vi "Save_to_Project.vi"(8 "error in (no error)":errorcluster, 9 "index in":string, 10 "buildObject":T2, 11 "IB_RegGroup in":refnum<class "IB_RegGroup.lvclass">) -> (0 "error out":errorcluster, 1 "index out":string, 2 "buildObject out":T2, 3 "IB_RegGroup out":refnum<class "IB_RegGroup.lvclass">)   [LabVIEW 2020, in "IB_RegGroup.lvclass"]
uses:
  <vilib>/AppBuilder/IB_Classes/RegGroup/IB_RegGroup.lvclass
  <vilib>/AppBuilder/IB_Classes/RegGroup/IB_RegGroup.lvclass/IB_RegGroup.ctl
  <vilib>/AppBuilder/IB_Classes/RegData/IB_RegData.lvclass
  <vilib>/AppBuilder/IB_RW_Project/IB_RW_Project_PropBag_Action.ctl
  <resource>/Framework/Providers/API/ItemRef.ctl
  <vilib>/AppBuilder/IB_RW_Project/IB_RW_Project_RegGroup_Data.ctl
panel:
  in  "RegGroup":T1
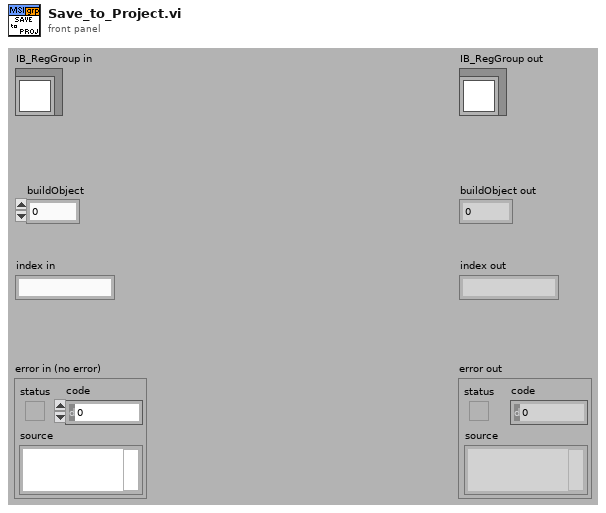
[diagram p1: front panel]
types:
  T1 = typedef "IB_RW_Project_RegGroup_Data.ctl" = cluster{"dirTag":string}
  T2 = typedef "ItemRef.ctl" = u64
  T3 = typedef "IB_RW_Project_PropBag_Action.ctl" = enum16{"read", "write", "clear", "readPrevious", "writePrevious", "clearPrevious"}
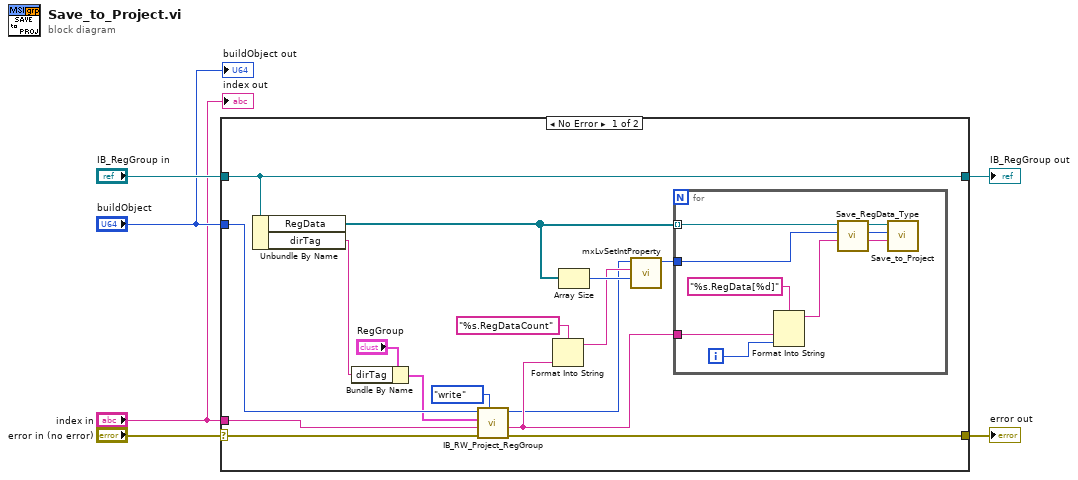
[diagram p0: block diagram]
diagram:
  n1 = case shown="No Error" "error in (no error)" {
    selector: "error in (no error)" -> [w16 w33]
    tunnel: [w15 w33] -> w5
    tunnel: [w18 w32] -> w3
    tunnel: "IB_RegGroup in" -> [w18 w32]
    tunnel: "buildObject" -> [w13 _]
    tunnel: "index in" -> [w12 _]
    frame No Error {
      n2 = Unbundle By Name(w18) -> ("RegData"=w17:refnum<class "IB_RegData.lvclass">[], "dirTag"=w8:string)
      n3 = Bundle By Name(cluster="RegGroup", "dirTag"=w8) -> (w7:T1)
      n4 = call <vilib>:"IB_RW_Project_RegGroup.vi"("action"=IB_RW_Project_PropBag_Action."write", "error in (no error)"=w16, "index in"=w12, "RegGroup"=w7, "buildObject"=w13) -> ("error out"=w15:errorcluster, "index out"=w11:string, "buildObject out"=w10:T2)  [unwired: 3 in, 1 out]
      n5 = Format Into String(format string="%s.RegDataCount", w11) -> (resulting string=w21:string)  [unwired: 2 in, 1 out]
      n6 = Array Size(array=w17) -> (size(s)=w22:i32)
      n7 = call <resource>:"mxLvSetIntProperty.vi"("Value (0)"=w22, "Tag"=w21, "Item"=w10) -> ("Item"=w19:T2)  [unwired: 7 in, 1 out]
      n8 = for {
        tunnel: w17 -> [w28] mode=indexing
        tunnel: w19 -> [w26]
        tunnel: w11 -> [w30]
        i -> [w29]
        n9 = Format Into String(format string="%s.RegData[%d]", w30, w29) -> (resulting string=w24:string)  [unwired: 2 in, 1 out]
        n10 = call-dynamic "Save_RegData_Type.vi"("index in"=w24, "buildObject"=w26, "IB_RegData in"=w28) -> ("index out"=w23:string, "buildObject out"=w25:T2, "IB_RegData out"=w27:refnum<class "IB_RegData.lvclass">)  [unwired: 5 in, 1 out]
        n11 = call-dynamic "Save_to_Project.vi"("index in"=w23, "buildObject"=w25, "IB_RegData in"=w27) -> ()  [unwired: 5 in, 4 out]
      }
    }
    frame Error {
    }
  }
  "error out" <- w5
  "IB_RegGroup out" <- w3
  "buildObject out" <- "buildObject"
  "index out" <- "index in"
